vi "DisconnectUDP.vi"(11 "FPGA in":refnum<queue>) -> (3 "FPGA out":refnum<queue>)   [LabVIEW 2019, in "FPGA.lvlib"]
uses:
  FPGA.lvlib
  FPGA.ctl
panel:
  out "Disconnected":bool
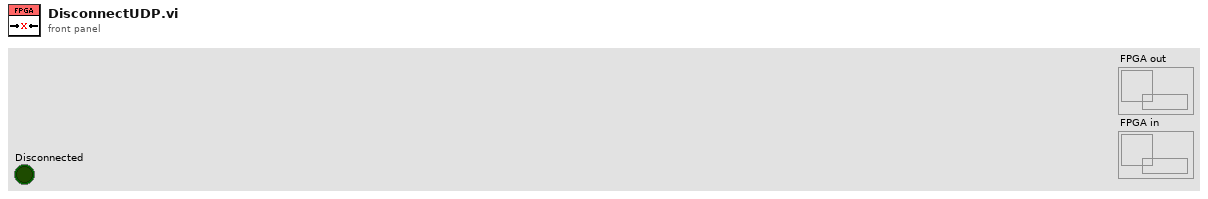
[diagram p1: front panel]
types:
  T1 = typedef "FPGA.lvlib/FPGA.ctl" = cluster{"Start freq. [Hz]":dbl, "Sweep duration [s]":dbl, "Freq. step [Hz]":dbl, "DAC Sample Rate":dbl, "ADC Sample Rate":dbl, "CMD port":u16, "DFAST port":u16, "CMD ID":refnum<k16>, "DFAST ID":refnum<k16>, "CMD error out":errorcluster, "FPGA IP":string, "DFAST error out ":errorcluster, "Stop freq. [Hz]":dbl, "Discrete sweep":bool, "Initial NCO":u32, "Difference NCO":i32, "step NCO":i64, "Final NCO":u32, "clocks for step":u32, "demodulation":bool, "NCO Phase Precision":u32, "NCO Sample Rate":dbl, "Time for step [s]":dbl, "NCO freq. resolution":dbl, "Sweep speed [Hz/s]":dbl, "Connected":bool, "Slew Rate [V/us]":dbl, "Parameters_ok":bool, "Amplitude [mVpp]":dbl, "Scale Factor":fxp<+,16,0>, "Acquiring":bool, "DAC-ADC Latency":u16, "Digital Gain":i32, "Number of steps":i32, "Averaging preferred":bool, "Filter Order":u32, "Settling":enum16{"99%", "99,9%"}}
  T2 = cluster{"[0]":errorcluster, "[1]":errorcluster, "[2]":errorcluster, "[3]":errorcluster}
  T3 = cluster{"[0]":refnum<k16>, "[1]":refnum<k16>, "[2]":refnum<k16>, "[3]":refnum<k16>}
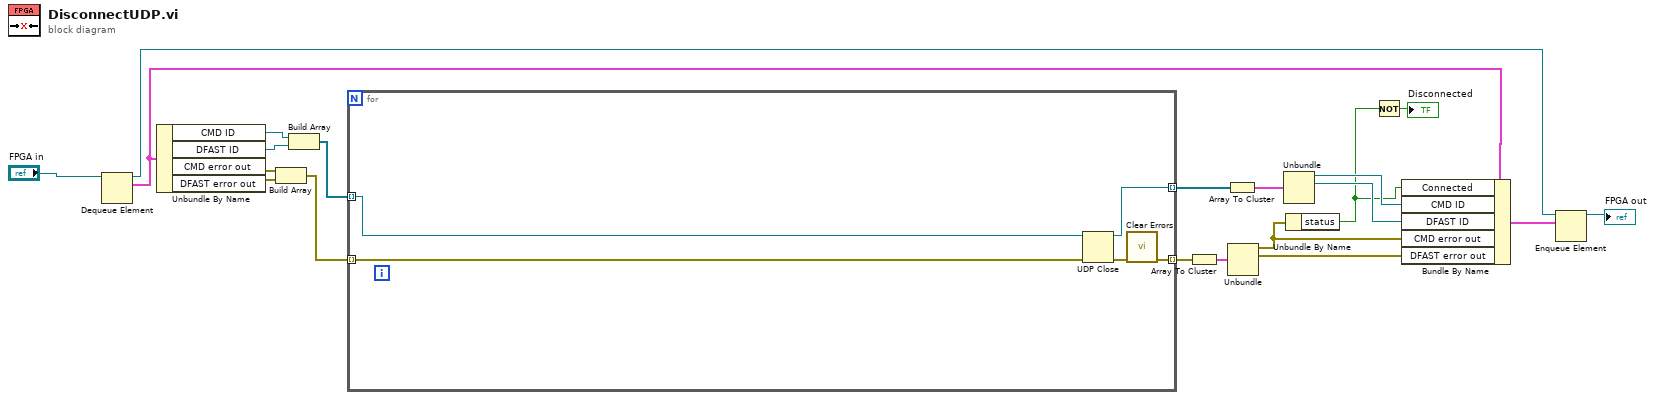
[diagram p0: block diagram]
diagram:
  n1 = Dequeue Element(queue="FPGA in") -> (queue out=w21:refnum<queue>, element=w17:T1)  [unwired: 2 in, 2 out]
  n2 = Unbundle By Name(w17) -> ("CMD ID"=w19:refnum<k16>, "DFAST ID"=w18:refnum<k16>, "CMD error out"=w15:errorcluster, "DFAST error out"=w14:errorcluster)
  n3 = Build Array(w15, w14) -> (w12:errorcluster[])
  n4 = Build Array(w19, w18) -> (w13:refnum<k16>[])
  n5 = for {
    tunnel: w13 -> [w25] mode=indexing
    tunnel: w12 -> [w24] mode=indexing
    tunnel: [w26] -> w10 mode=indexing
    tunnel: [w22] -> w11 mode=indexing
    n6 = UDP Close(connection ID=w25, 8:w24) -> (connection ID out=w22:refnum<k16>, error out=w23:errorcluster)
    n7 = call <vilib>:"Clear Errors.vi"("error in (no error)"=w23) -> ("error out"=w26:errorcluster)  [unwired: 5 in, 1 out]
  }
  n8 = Array To Cluster(array=w10) -> (cluster=w8:T2)
  n9 = Array To Cluster(array=w11) -> (cluster=w9:T3)
  n10 = Unbundle(w8) -> ("[0]"=w4:errorcluster, "[1]"=w7:errorcluster)  [unwired: 2 out]
  n11 = Unbundle(w9) -> ("[0]"=w5:refnum<k16>, "[1]"=w6:refnum<k16>)  [unwired: 2 out]
  n12 = Unbundle By Name(w4) -> ("status"=w2:bool)
  n13 = Not(x=w2) -> (.not. x?=→"Disconnected":bool)
  n14 = Bundle By Name(cluster=w17, "Connected"=w2, "CMD ID"=w5, "DFAST ID"=w6, "CMD error out"=w4, "DFAST error out"=w7) -> (w20:T1)
  n15 = Enqueue Element(queue=w21, element=w20) -> (queue out=→"FPGA out":refnum<queue>)  [unwired: 2 in, 2 out]
